vi "04 - Exemple - AsyncRepeatSum.vi"() -> ()   [LabVIEW 2016]
uses:
  Library/DemoSkeleton/DemoSkeleton.lvlib
panel:
  in  "stop":bool
  in  "B":i32=2
  in  "A":i32=1
  out "Sum":i64
  # "+"
  # "="
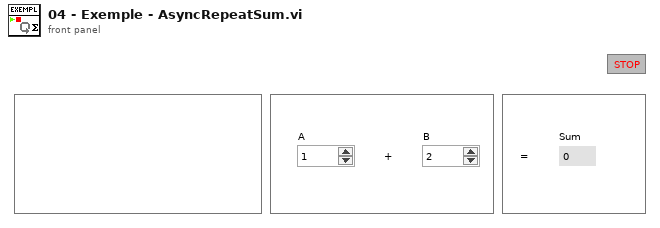
[diagram p1: front panel]
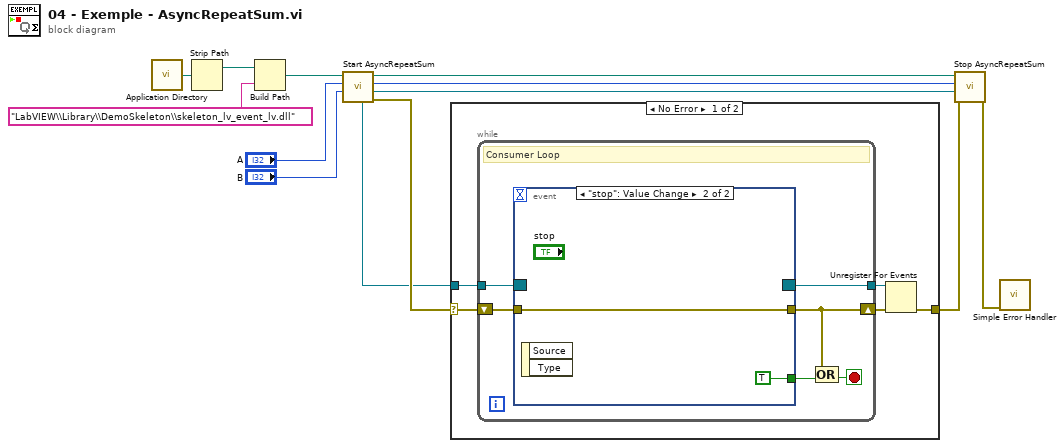
[diagram p0: block diagram]
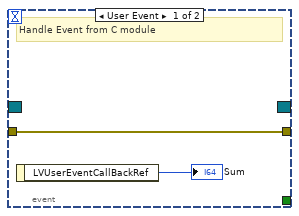
[diagram p2: hidden frame]
diagram:
  n1 = call <vilib>:"Application Directory.vi"() -> ("Application Directory"=w4:path)
  n2 = Strip Path(path=w4) -> (stripped path=w3:path)  [unwired: 1 out]
  n3 = Build Path(base path=w3, name or relative path="LabVIEW\\Library\\DemoSkeleton\\skeleton_lv_event_lv.dll") -> (appended path=w1:path)
  n4 = call "Start AsyncRepeatSum.vi"("B"="B", "A"="A", "path in"=w1) -> ("error out"=w13:errorcluster, "LVUserEvent CallBack Reference"=w6:refnum<user-event>, "Handle"=w11:u64, "dup path"=w12:path, "AsyncSum Event Register"=w5:refnum<event-registration>)  [unwired: 4 in]
  n5 = case shown="No Error" w13 {
    selector: w13 -> [w16 w29]
    tunnel: w5 -> [w15 _]
    tunnel: [w14 w29] -> w10
    frame No Error {
      n6 = while {
        shift-right: [w21] -> w17
        shift-left: w16 -> [w23]
        tunnel: w15 -> [w22]
        tunnel: [w24] -> w18
        stop <- w20 stop-if-true
        # "Consumer Loop"
        n7 = event shown="[1] \"stop\": Value Change" {
          selector: w22 -> [_ _]
          dyn-events: [_ _] -> w24
          timeout: _ -> [_ _]
          tunnel: w23 -> [w26 w28]
          tunnel: [w26 w28] -> w21
          tunnel: [_ TRUE] -> w19
          event User Event {
            # "Handle Event from C module"
            n8 = event-data() -> ("LVUserEventCallBackRef"=→"Sum":i64)  [unwired: 1 in]
          }
          event "stop": Value Change {
            n9 = event-data() -> ()  [unwired: 1 in, 2 out]
          }
        }
        n10 = Compound Arithmetic op=OR(w21, w19) -> (w20:bool)
      }
      n11 = Unregister For Events(event registration refnum=w18, error in=w17) -> (error out=w14:errorcluster)
    }
    frame Error {
    }
  }
  n12 = call "Stop AsyncRepeatSum.vi"("error in (no error)"=w10, "LVUserEventCallBackRef"=w6, "Handle"=w11, "path in"=w12) -> ("error out"=w9:errorcluster)  [unwired: 6 in, 1 out]
  n13 = call <vilib>:"Simple Error Handler.vi"("error in (no error)"=w9) -> ()  [unwired: 4 in, 5 out]
